vi "Init.vi"(4 "Interlock message (\" -> Interlock!\")":string=" -> Interlock!", 6 "Name (SHV Name if empty)":string, 7 "SHV":variant, 8 "error in (no error)":errorcluster, 9 "Stop Self on IL? (T)":bool=TRUE, 11 "Interlock in":refnum<class "Interlock.lvclass">) -> (0 "error out":errorcluster, 3 "Interlock out":refnum<class "Interlock.lvclass">)   [LabVIEW 2015, in "Interlocks.lvlib" / "Interlock.lvclass"]
uses:
  Interlock.lvclass
  Interlock.lvclass/Interlock.ctl
  <vilib>/ActorFramework/Message Enqueuer/Message Priority.ctl
  IL Action/IL Action.lvclass
  <vilib>/ActorFramework/Message Enqueuer/Message Enqueuer.lvclass
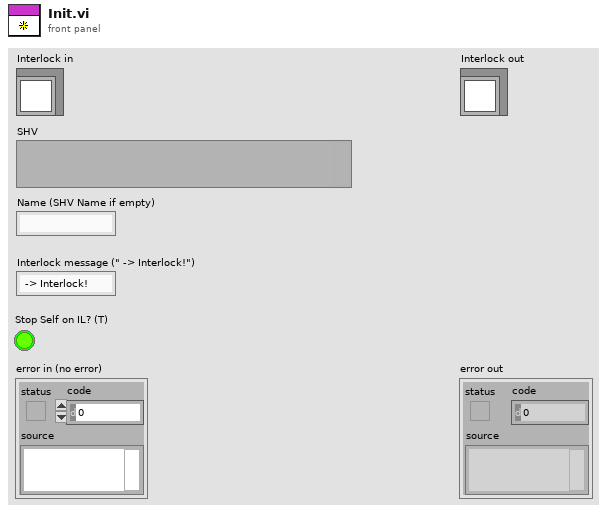
[diagram p1: front panel]
types:
  T1 = cluster{"Read Access":enum8{"Allowed", "Required", "None"}, "Write Access":enum8{"Allowed", "Required", "None"}}
  T2 = typedef "Actor Framework.lvlib/Message Enqueuer.lvclass/Message Priority.ctl" = enum16{"Low", "Normal", "High"}
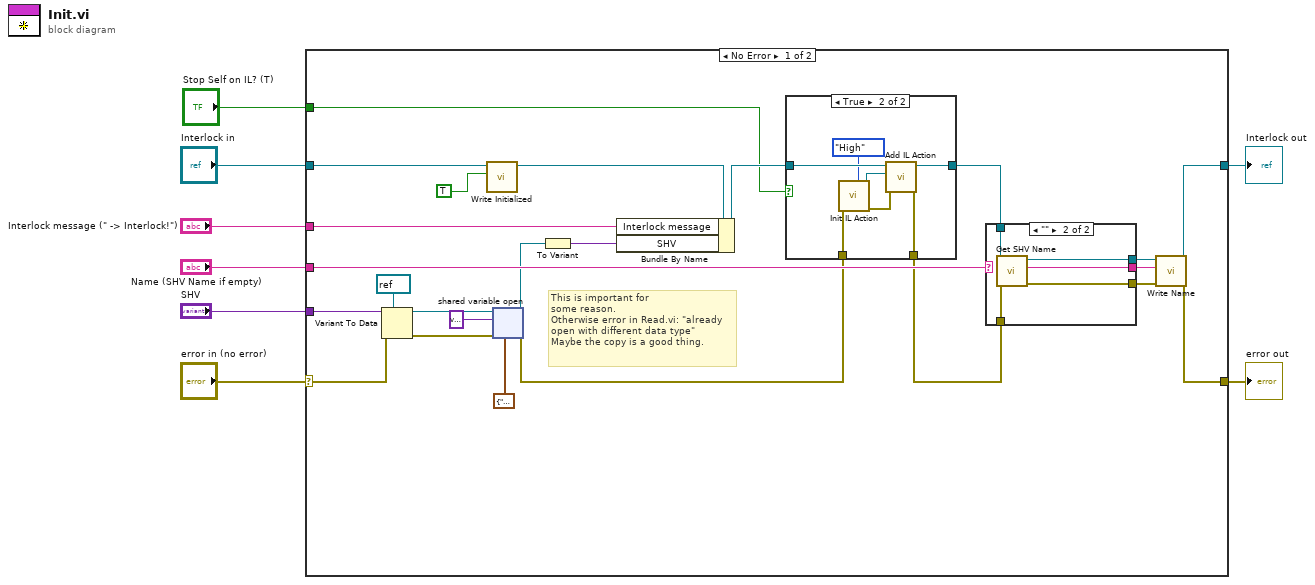
[diagram p0: block diagram]
diagram:
  n1 = case shown="No Error" "error in (no error)" {
    selector: "error in (no error)" -> [w18 w51]
    tunnel: [w26 w51] -> w7
    tunnel: [w25 w50] -> w5
    tunnel: "Interlock in" -> [w32 w50]
    tunnel: "SHV" -> [w16 _]
    tunnel: "Name (SHV Name if empty)" -> [w24 _]
    tunnel: "Interlock message (\" -> Interlock!\")" -> [w23 _]
    tunnel: "Stop Self on IL? (T)" -> [w9 _]
    frame No Error {
      # "This is important for\nsome reason.\nOtherwise error in Read.vi: \"already\nopen with different data type\"\nMaybe the copy is a good thing."
      n2 = Variant To Data(error in=w18, type=refnum<k21> refnum ("SHV"), Variant=w16) -> (data=w17:refnum<k21>, error out=w19:errorcluster)
      n3 = call-dynamic "Write Initialized.vi"("Initialized (True)"=TRUE ("Initialized"), "Interlock in"=w32) -> ("Interlock out"=w15:refnum<class "Interlock.lvclass">)  [unwired: 9 in]
      n4 = shared-variable-open(w17, w19, variant ("variant"), T1 {"Read Access"=enum."Allowed", "Write Access"=enum."None"} ("access")) -> (w22:refnum<k21>, w11:errorcluster)
      n5 = To Variant(anything=w22) -> (Variant=w21:variant)
      n6 = Bundle By Name(cluster=w15, "Interlock message"=w23, "SHV"=w21) -> (w13:refnum<class "Interlock.lvclass">)
      n7 = case shown="True" w9 {
        tunnel: w13 -> [w33 w41]
        tunnel: [w33 w40] -> w12
        tunnel: w11 -> [w34 w38]
        tunnel: [w34 w39] -> w10
        frame False {
        }
        frame True {
          n8 = call "Init IL Action.vi"("Message Priority (Normal)"=Message_Priority."High", "error in (no error)"=w38) -> ("error out"=w37:errorcluster, "IL Action out"=w36:refnum<class "IL Action.lvclass">)  [unwired: 8 in]
          n9 = call "Add IL Action.vi"("error in (no error)"=w37, "IL Action in"=w36, "Interlock in"=w41) -> ("error out"=w39:errorcluster, "Interlock out"=w40:refnum<class "Interlock.lvclass">)  [unwired: 7 in]
        }
      }
      n10 = case shown="\"\"" w24 {
        selector: w24 -> [w44 _]
        tunnel: [w44 w49] -> w29
        tunnel: [w43 w48] -> w28
        tunnel: w10 -> [w42 w47]
        tunnel: [w42 w46] -> w27
        tunnel: w12 -> [w43 w45]
        frame "False", Default {
        }
        frame "" {
          n11 = call "Get SHV Name.vi"("error in (no error)"=w47, "Interlock in"=w45) -> ("error out"=w46:errorcluster, "Name"=w49:string, "Interlock out"=w48:refnum<class "Interlock.lvclass">)  [unwired: 7 in]
        }
      }
      n12 = call "Write Name.vi"("error in (no error)"=w27, "Name"=w29, "Interlock in"=w28) -> ("error out"=w26:errorcluster, "Interlock out"=w25:refnum<class "Interlock.lvclass">)  [unwired: 7 in]
    }
    frame Error {
    }
  }
  "error out" <- w7
  "Interlock out" <- w5
